vi "Compute Indegrees.vi"(8 "error in (no error)":errorcluster, 11 "Topological Sort in":refnum<class "Topological Sort.lvclass">) -> (0 "error out":errorcluster, 3 "Topological Sort out":refnum<class "Topological Sort.lvclass">)   [LabVIEW 2025, in "AOC.lvlib" / "Topological Sort.lvlib" / "Topological Sort.lvclass"]
uses:
  Topological Sort.lvclass
  Topological Sort.lvclass/Topological Sort.ctl
  Graph/Graph.lvclass
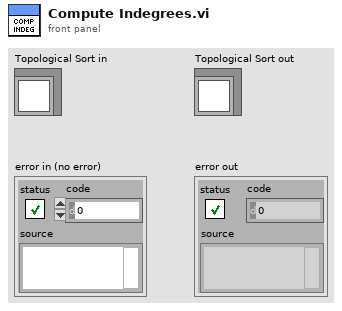
[diagram p1: front panel]
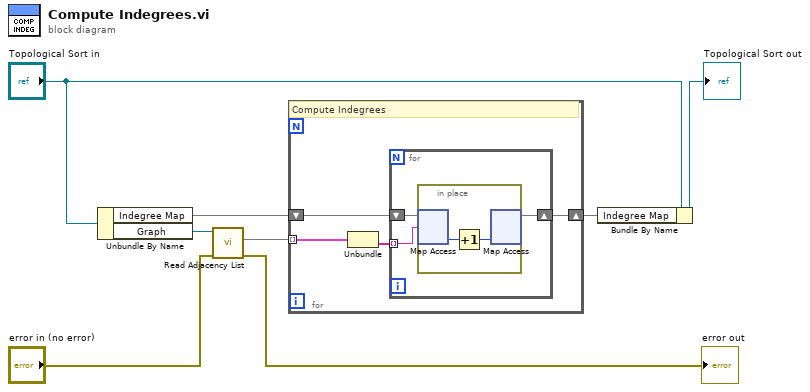
[diagram p0: block diagram]
diagram:
  n1 = Unbundle By Name("Topological Sort in") -> ("Indegree Map"=w3:map{string, u64}, "Graph"=w7:refnum<class "Graph.lvclass">)
  n2 = call-dynamic "Read Adjacency List.vi"("error in (no error)"="error in (no error)", "Graph in"=w7) -> ("error out"=→"error out":errorcluster, "Adjacency List"=w6:map{string, string[]})  [unwired: 7 in, 1 out]
  n3 = for {
    tunnel: w6 -> [w12] mode=indexing
    shift-right: [w10] -> w1
    shift-left: w3 -> [w11]
    # "Compute Indegrees"
    n4 = Unbundle(w12) -> (w9:string[])  [unwired: 1 out]
    n5 = for {
      tunnel: w9 -> [w13] mode=indexing
      shift-right: [w14] -> w10
      shift-left: w11 -> [w15]
      n6 = in-place {
        n7 = in-place-map #1(w15, w13) -> (w17:u64)  [unwired: 1 in, 1 out]
        n8 = Increment(x=w17) -> (x+1=w16:u64)
        n9 = in-place-map #1(w16) -> (w14:map{string, u64})  [unwired: 1 in, 2 out]
      }
    }
  }
  n10 = Bundle By Name(cluster="Topological Sort in", "Indegree Map"=w1) -> (→"Topological Sort out":refnum<class "Topological Sort.lvclass">)
